vi "Extract Icon Data.vi"(7 "Text layer name":string="Text", 10 "Icon data in":T1={"Text Visible?"=FALSE, "Text Opacity"=0, "Templ Visible?"=FALSE, "Templ Opacity"=0, "Relative Path from 1 to 2"=path "", "Image"=bytes[0], "All User Layers"=[], "Body Text"={"Line 1 text"="", "Line 2 text"="", "Line 3 text"="", "Line 4 text"="", "Line 1 color"=0, "Line 2 color"=0, "Line 3 color"=0, "Line 4 color"=0, "Body Text Spec"={"Font"="", "Alignment"=0, "Size"=3}, "Center text vertically"=FALSE, "Capitalize Text"=FALSE}} {"Body Text"."Body Text Spec"."Alignment" items=["left", "center", "right"]}, 11 "Template layer name":string="Template") -> (1 "Template data":T5={"LayerIcon"=bytes[3230], "LayerName"="Template", "Opacity"=100, "Visibility?"=TRUE} {"Opacity" scale=0.0..100.0}, 2 "Icon data out":T1={"Text Visible?"=FALSE, "Text Opacity"=0, "Templ Visible?"=FALSE, "Templ Opacity"=0, "Relative Path from 1 to 2"=path "", "Image"=bytes[0], "All User Layers"=[], "Body Text"={"Line 1 text"="", "Line 2 text"="", "Line 3 text"="", "Line 4 text"="", "Line 1 color"=0, "Line 2 color"=0, "Line 3 color"=0, "Line 4 color"=0, "Body Text Spec"={"Font"="", "Alignment"=0, "Size"=3}, "Center text vertically"=FALSE, "Capitalize Text"=FALSE}} {"Body Text"."Body Text Spec"."Alignment" items=["left", "center", "right"]}, 3 "Text data":T5={"LayerIcon"=bytes[0], "LayerName"="", "Opacity"=100, "Visibility?"=TRUE} {"Opacity" scale=0.0..100.0}, 4 "Active template (faked Array)":T6={"Rectangle"={"left"=0, "top"=0, "right"=0, "bottom"=0}, "Path"=path "", "Image"=bytes[3230], "Filter"="", "FileName"=""})   [LabVIEW 2020, in "LabVIEW Icon API.lvlib"]
doc: "Extract the actual LabVIEW Icon Data."
uses:
  <vilib>/LabVIEW Icon API/LabVIEW Icon API.lvlib
  <vilib>/LabVIEW Icon API/lv_icon/Controls/Graphic.ctl
  <vilib>/LabVIEW Icon API/lv_icon/Controls/Layer.ctl
  <vilib>/LabVIEW Icon API/lv_icon/Controls/LabVIEW Icon Stored Information.ctl
  <vilib>/LabVIEW Icon API/lv_icon/Classes/Layer/Layer.lvclass
  <vilib>/LabVIEW Icon API/lv_icon/Controls/BodyText.ctl
  <vilib>/LabVIEW Icon API/lv_icon/Controls/Font.ctl
  <vilib>/LabVIEW Icon API/lv_icon/Controls/Alignment.ctl
  <vilib>/LabVIEW Icon API/lv_icon/lv_icon.lvlib
panel:
  in  "Loc":string="LabVIEW Icon API"
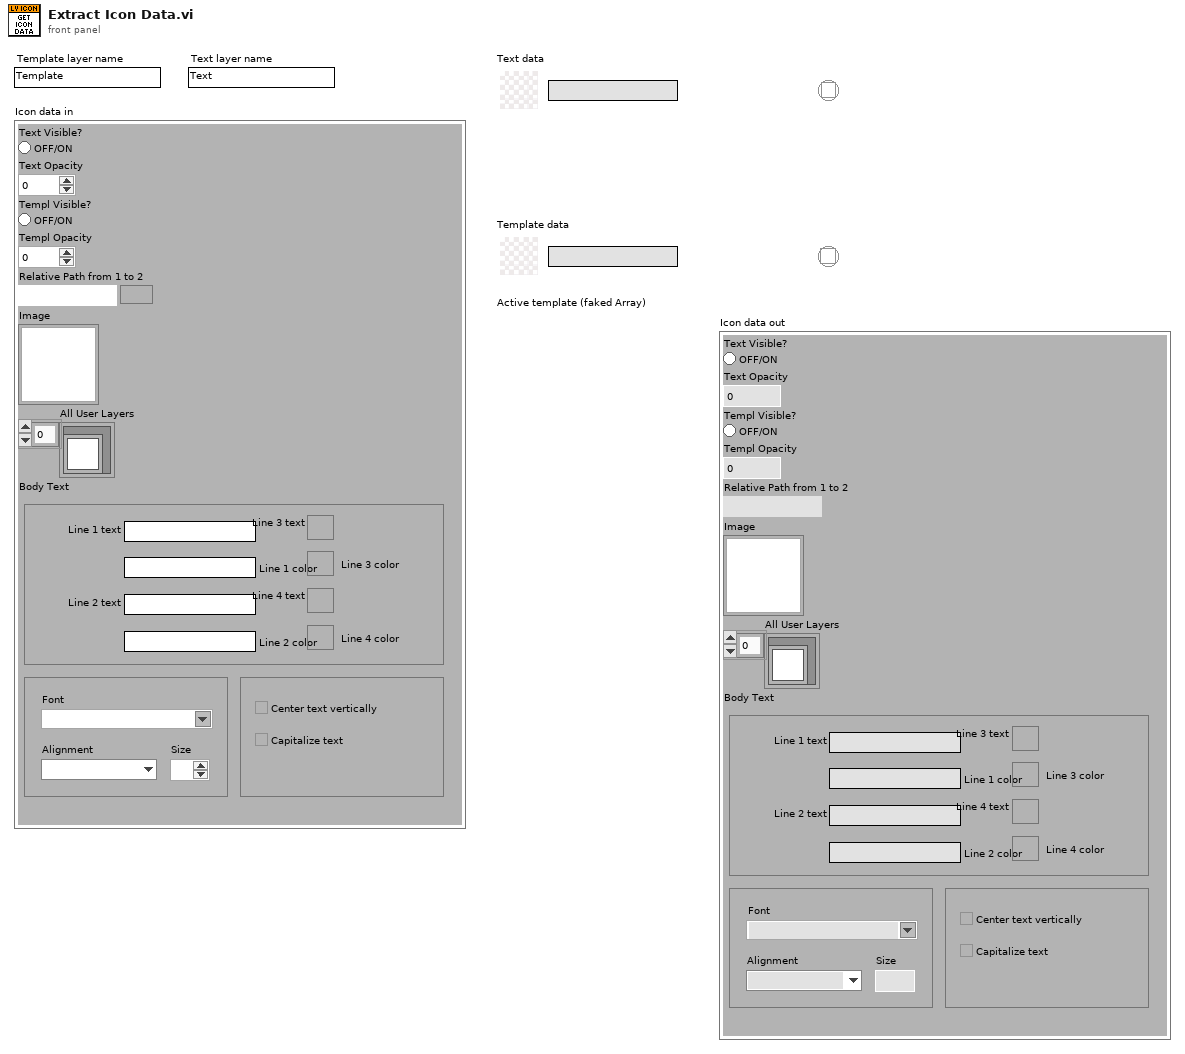
[diagram p1: front panel]
types:
  T1 = typedef "LabVIEW Icon Stored Information.ctl" = cluster{"Text Visible?":bool, "Text Opacity":u8, "Templ Visible?":bool, "Templ Opacity":u8, "Relative Path from 1 to 2":path, "Image":picture, "All User Layers":refnum<class "Layer.lvclass">[], "Body Text":T2}
  T2 = typedef "BodyText.ctl" = cluster{"Line 1 text":string, "Line 2 text":string, "Line 3 text":string, "Line 4 text":string, "Line 1 color":u32, "Line 2 color":u32, "Line 3 color":u32, "Line 4 color":u32, "Body Text Spec":cluster{"Font":T3, "Alignment":T4, "Size":u8}, "Center text vertically":bool, "Capitalize Text":bool}
  T3 = typedef "Font.ctl" = string
  T4 = typedef "Alignment.ctl" = u16
  T5 = typedef "Layer.ctl" = cluster{"LayerIcon":picture, "LayerName":string, "Opacity":u8, "Visibility?":bool}
  T6 = typedef "Graphic.ctl" = cluster{"Rectangle":cluster{"left":i16, "top":i16, "right":i16, "bottom":i16}, "Path":path, "Image":picture, "Filter":string, "FileName":string}
  T7 = typedef "imagedata.ctl" = cluster{"image type":i32, "image depth":i32, "image":u8[], "mask":u8[], "colors":u32[], "Rectangle":cluster{"left":i16, "top":i16, "right":i16, "bottom":i16}}
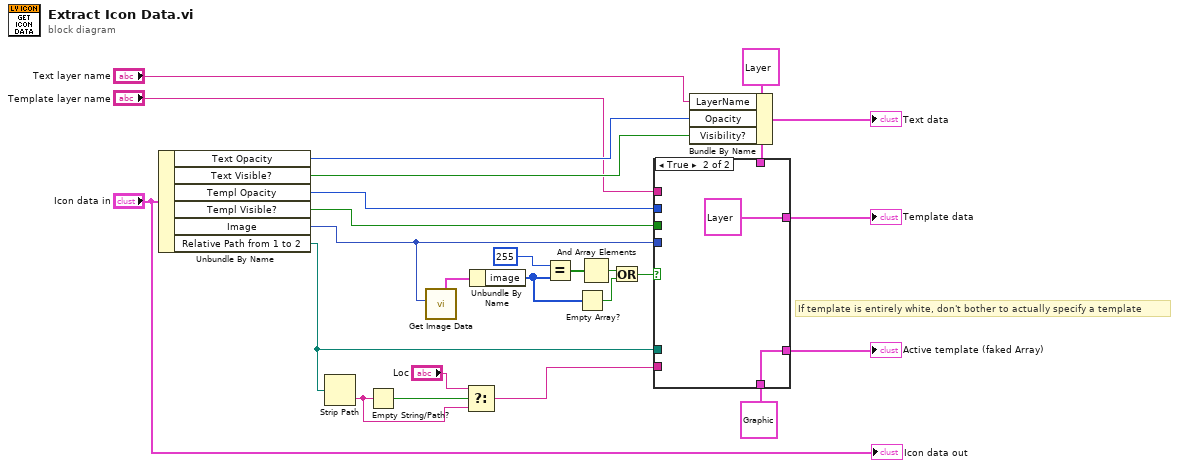
[diagram p0: block diagram]
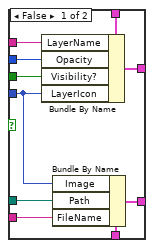
[diagram p2: hidden frame]
diagram:
  w1 = T5 {"LayerIcon"=bytes[0], "LayerName"="", "Opacity"=0, "Visibility?"=FALSE} ("Data")
  # "If template is entirely white, don't bother to actually specify a template"
  n1 = Unbundle By Name("Icon data in") -> ("Text Opacity"=w23:u8, "Text Visible?"=w22:bool, "Templ Opacity"=w17:u8, "Templ Visible?"=w18:bool, "Image"=w9:picture, "Relative Path from 1 to 2"=w19:path)
  n2 = Strip Path(path=w19) -> (name=w13:string)  [unwired: 1 out]
  n3 = Empty String/Path?(string/path=w13) -> (empty?=w10:bool)
  n4 = call <vilib>:"Get Image Data.vi"("Pic In"=w9) -> ("image data out"=w8:T7)  [unwired: 2 in, 8 out]
  n5 = Select(t="Loc", s=w10, f=w13) -> (s? t:f=w11:string)
  n6 = Unbundle By Name(w8) -> ("image"=w4:u8[])
  n7 = Equal?(x=u8 255, y=w4) -> (x = y?=w6:bool[])
  n8 = Empty Array?(array=w4) -> (empty?=w3:bool)
  n9 = And Array Elements(Boolean array=w6) -> (logical AND=w5:bool)
  n10 = Or(x=w5, y=w3) -> (x .or. y?=w2:bool)
  n11 = case shown="True" w2 {
    tunnel: [w35 w37] -> w25
    tunnel: T6 {"Rectangle"={"left"=0, "top"=0, "right"=0, "bottom"=0}, "Path"=path "", "Image"=bytes[0], "Filter"="", "FileName"=""} ("Path & Icon") -> [w34 w37]
    tunnel: [w33 T5 {"LayerIcon"=bytes[0], "LayerName"="", "Opacity"=0, "Visibility?"=FALSE} ("Data")] -> w20
    tunnel: w19 -> [w32 _]
    tunnel: w18 -> [w31 _]
    tunnel: w17 -> [w30 _]
    tunnel: "Template layer name" -> [w29 _]
    tunnel: w11 -> [w28 _]
    tunnel: w9 -> [w27 _]
    tunnel: w1 -> [w26 _]
    frame False {
      n12 = Bundle By Name(cluster=w26, "LayerName"=w29, "Opacity"=w30, "Visibility?"=w31, "LayerIcon"=w27) -> (w33:T5)
      n13 = Bundle By Name(cluster=w34, "Image"=w27, "Path"=w32, "FileName"=w28) -> (w35:T6)
    }
    frame True {
    }
  }
  "Active template (faked Array)" <- w25
  "Template data" <- w20
  n14 = Bundle By Name(cluster=w1, "LayerName"="Text layer name", "Opacity"=w23, "Visibility?"=w22) -> (→"Text data":T5)
  "Icon data out" <- "Icon data in"
